vi "oa_Decimation with CIC and Compensation Filter.vi"(0 "x[n]":dbl[](array[numeric]) format="%.2f", 1 "reset? (True)":bool=TRUE, 5 "CIC decimation setting":T2, 7 "decimation filters":T1[](array[typedef]) {"coefficients" format="%.2f"}, 11 "error in (no error)":errorcluster, 12 "statein":cluster{cluster{dbl[]}, cluster{dbl[]}[]}, 13 "interpolation factor":i32) -> (4 "x[n] out":dbl[](array[numeric]) format="%.2f", 14 "state out":cluster{cluster{dbl[]}, cluster{dbl[]}[]}, 15 "error out":errorcluster)   [LabVIEW 2017, in "SoundVib_Resampling.lvlib"]
uses:
  <vilib>/addons/Sound and Vibration/Order Analysis/Resample Order Tracking/SoundVib_Resampling.lvlib
  <vilib>/addons/_NISVFA/_Shared subVIs/Controls/OAT Decimation Filter.ctl
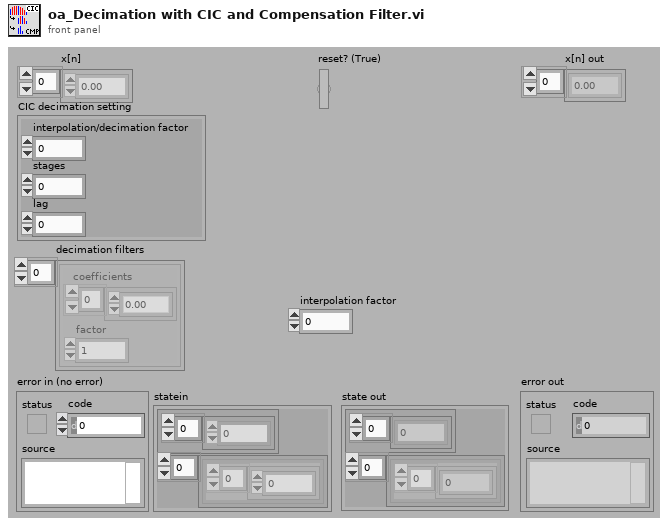
[diagram p1: front panel]
types:
  T1 = typedef "OAT Decimation Filter.ctl" = cluster{"coefficients":dbl[], "factor":i32}
  T2 = cluster{"interpolation/decimation factor":i32, "stages":i32, "lag":i32}
  T3 = cluster{"interpolation/decimation factor":i32, "stages":i32, "lag":i32}[]
  T4 = cluster{cluster{"final state":dbl[]}, cluster{"final state":dbl[]}[]}
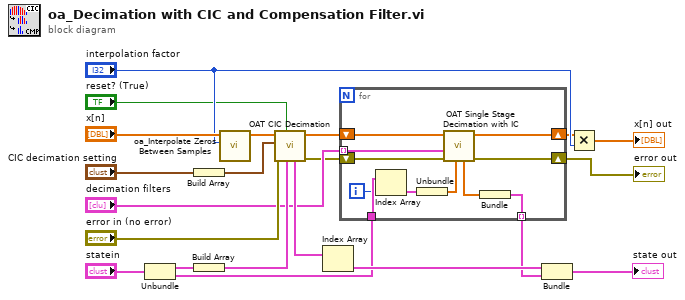
[diagram p0: block diagram]
diagram:
  n1 = Unbundle("statein") -> (w10:cluster{dbl[]}, w6:cluster{dbl[]}[])
  n2 = Build Array("CIC decimation setting") -> (w20:T3)
  n3 = Build Array(w10) -> (w16:cluster{dbl[]}[])
  n4 = call <vilib>:"oa_Interpolate Zeros Between Samples.vi"("interpolation factor"="interpolation factor", "x"="x[n]") -> ("x out"=w12:dbl[])  [unwired: 9 in]
  n5 = call <vilib>:"OAT CIC Decimation.vi"("initial state"=w16, "reset? (True)"="reset? (True)", "error in (no error)"="error in (no error)", "CIC filter settings"=w20, "X"=w12) -> ("error out"=w4:errorcluster, "Y"=w7:dbl[], "final state"=w18:cluster{"final state":dbl[]}[])  [unwired: 4 in]
  n6 = Index Array(array=w18) -> (element=w17:cluster{"final state":dbl[]})  [unwired: 1 in]
  n7 = for {
    tunnel: "decimation filters" -> [w32] mode=indexing
    shift-right: [w24] -> w3
    shift-left: w7 -> [w31]
    tunnel: w6 -> [w30]
    tunnel: [w25] -> w5 mode=indexing
    shift-right: [w22] -> w2
    shift-left: w4 -> [w23]
    i -> [w29]
    n8 = Index Array(array=w30, index=w29) -> (element=w28:cluster{dbl[]})
    n9 = Unbundle(w28) -> (w27:dbl[])
    n10 = call <vilib>:"OAT Single Stage Decimation with IC.vi"("initial state"=w27, "error in (no error)"=w23, "filter"=w32, "X"=w31) -> ("error out"=w22:errorcluster, "Y"=w24:dbl[], "final state"=w26:dbl[])  [unwired: 5 in]
    n11 = Bundle("final state"=w26) -> (w25:cluster{"final state":dbl[]})  [unwired: 1 in]
  }
  "error out" <- w2
  n12 = Bundle(w17, w5) -> (→"state out":T4)  [unwired: 1 in]
  n13 = Multiply(x=w3, y="interpolation factor") -> (x*y=→"x[n] out":dbl[])
